vi "CameraReadJPEGtoFile.vi"(8 "error in":errorcluster, 11 "IO Cluster In":T1={"Error"={"status"=FALSE, "code"=0, "source"=""}, "Encoder Calibration Values"=[22, 216], "Update Calibration"=FALSE, "JPEG Resolutions"=3, "Raw Resolutions"=1, "Image Mode"=enum."RAW Gray Scale", "FPGA Ref"=refnum} {"JPEG Resolutions" items=["160x128"=3, "320x240"=5, "640x480"=7]; "Raw Resolutions" items=["80x60"=1, "160x120"=3, "128x128"=9, "128x96"=11]}) -> (0 "Error Out":errorcluster, 1 "Image File":path=path "/home/lvuser/natinst/bin/CamImage.jpg", 2 "New Image Data":bool, 3 "IO Cluster Out":T1={"Error"={"status"=FALSE, "code"=0, "source"=""}, "Encoder Calibration Values"=[22, 216], "Update Calibration"=FALSE, "JPEG Resolutions"=3, "Raw Resolutions"=1, "Image Mode"=enum."RAW Gray Scale", "FPGA Ref"=refnum} {"JPEG Resolutions" items=["160x128"=3, "320x240"=5, "640x480"=7]; "Raw Resolutions" items=["80x60"=1, "160x120"=3, "128x128"=9, "128x96"=11]})   [LabVIEW 2018]
uses:
  QNET MS IO Cluster.ctl
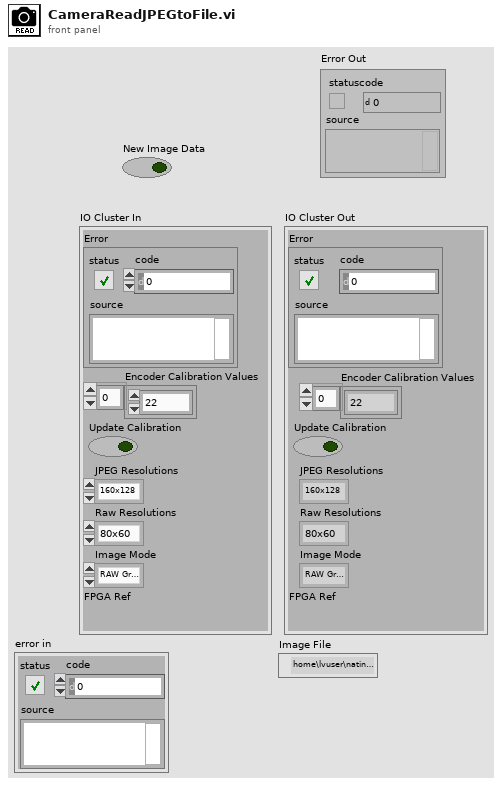
[diagram p1: front panel]
types:
  T1 = typedef "QNET MS IO Cluster.ctl" = cluster{"Error":errorcluster, "Encoder Calibration Values":i32[], "Update Calibration":bool, "JPEG Resolutions":u16, "Raw Resolutions":u16, "Image Mode":enum16{"RAW RGB", "RAW Gray Scale", "JPEG"}, "FPGA Ref":refnum<k20>}
  T2 = enum16{"big-endian, network order", "native, host order", "little-endian"}
  T3 = enum16{"open", "replace", "create", "open or create", "replace or create", "replace or create with confirmation"}
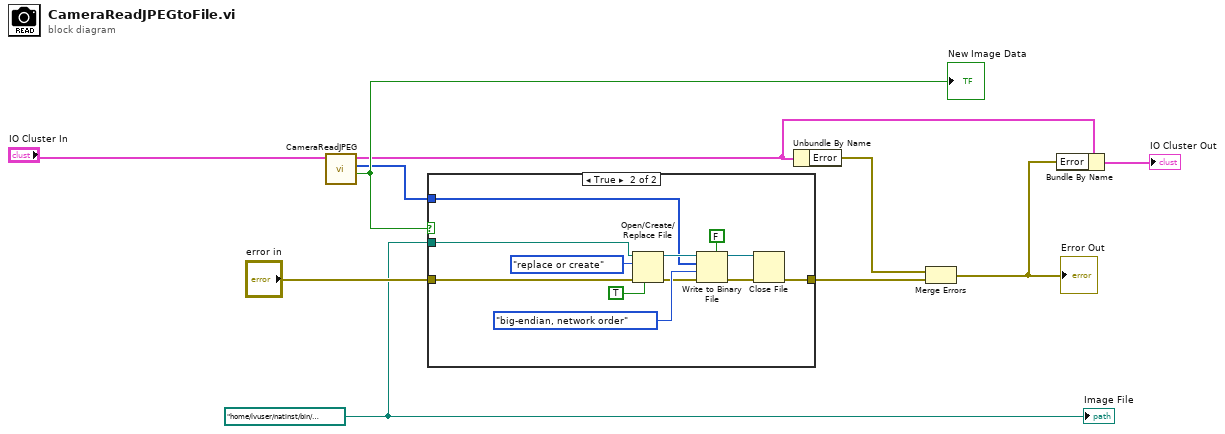
[diagram p0: block diagram]
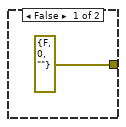
[diagram p2: hidden frame]
diagram:
  w1 = path "/home/lvuser/natinst/bin/CamImage.jpg" ("file path (use dialog)")
  n1 = call "CameraReadJPEG.vi"("IO Cluster In"="IO Cluster In") -> ("New Image Data"=w10:bool, "Image Data"=w6:u8[], "IO Cluster Out"=w9:T1)  [unwired: 6 in, 2 out]
  "New Image Data" <- w10
  n2 = case shown="True" w10 {
    tunnel: w6 -> [_ w15]
    tunnel: [errorcluster {"status"=FALSE, "code"=0, "source"=""} ("error out") w14] -> w5
    tunnel: w1 -> [_ w13]
    tunnel: "error in" -> [_ w12]
    frame False {
    }
    frame True {
      n3 = Open/Create/Replace File(file path (use dialog)=w13, error in=w12, operation (0:open)=T3."replace or create", disable buffering (F)=TRUE) -> (refnum out=w18:refnum<file>, error out=w20:errorcluster)  [unwired: 2 in, 1 out]
      n4 = Write to Binary File(file (use dialog)=w18, data=w15, error in=w20, 5:FALSE ("prepend array or string size? (T)"), 9:T2."big-endian, network order" ("byte order (0:big-endian, network order)")) -> (refnum out=w19:refnum<file>, error out=w21:errorcluster)  [unwired: 1 in, 1 out]
      n5 = Close File(refnum=w19, error in=w21) -> (error out=w14:errorcluster)  [unwired: 1 out]
    }
  }
  n6 = Unbundle By Name(w9) -> ("Error"=w4:errorcluster)
  n7 = Merge Errors(w4, w5) -> (w3:errorcluster)
  "Error Out" <- w3
  n8 = Bundle By Name(cluster=w9, "Error"=w3) -> (→"IO Cluster Out":T1)
  "Image File" <- w1
